vi "Gripper Drive.vi"(7 "Description":string, 8 "Command Info In":T1, 11 "Right Motor":dbl) -> (0 "Command Info Out":T1)   [LabVIEW 2017]
doc: "This template is useful for immediate subsystem actions that do not need deadband filtering\n\nBe sure to right-click and select New from Template and save with a new command name."
uses:
  <vilib>/Rock Robotics/WPI/Framework/Command Status Info.ctl
  <vilib>/Rock Robotics/WPI/Framework/Completion Status.ctl
  <vilib>/Rock Robotics/WPI/Framework/Completion Notifier.ctl
  Implementation/Gripper Setpoints.ctl
  Implementation/Gripper Operations.ctl
  Left Setpoint.ctl
panel:
  in  "Left Motor":dbl
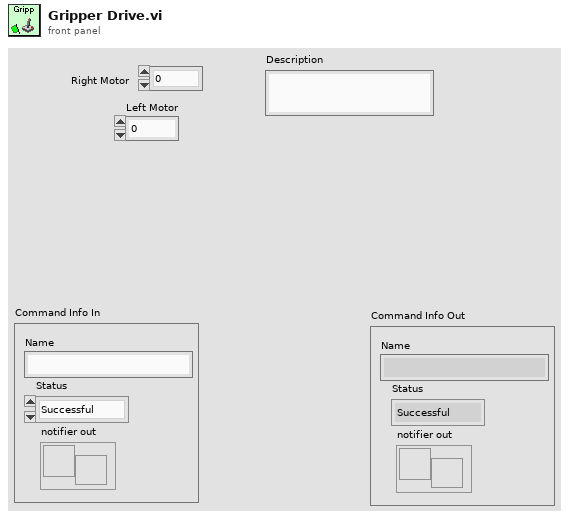
[diagram p1: front panel]
types:
  T1 = typedef "Command Status Info.ctl" = cluster{"Name":string, "Status":T2, "notifier out":T3}
  T2 = typedef "Completion Status.ctl" = enum16{"Successful", "Aborted", "Incomplete"}
  T3 = typedef "Completion Notifier.ctl" = refnum<notifier>
  T4 = typedef "Gripper Setpoints.ctl" = cluster{"Operation":T5, "Right Motor":T6, "Duration":dbl, "Left Motor":dbl}
  T5 = typedef "Gripper Operations.ctl" = enum16{"Reserve", "Read Current", "Immediate", "Set Gripper Motors"}
  T6 = typedef "Left Setpoint.ctl" = dbl
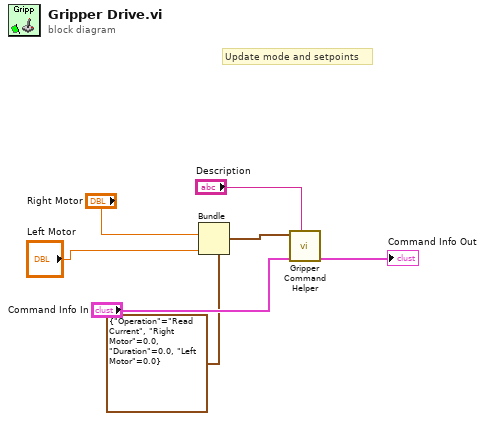
[diagram p0: block diagram]
diagram:
  # "Update mode and setpoints"
  n1 = Bundle(cluster=T4 {"Operation"=enum."Read Current", "Right Motor"=0.0, "Duration"=0.0, "Left Motor"=0.0} ("SubSystem Data"), "Right Motor"="Right Motor", "Left Motor"="Left Motor") -> (w2:T4)  [unwired: 2 in]
  n2 = call "Gripper Command Helper.vi"("Description"="Description", "Command Info In"="Command Info In", "SubSystem Data"=w2) -> ("Command Info Out"=→"Command Info Out":T1)  [unwired: 6 in, 2 out]
